vi "Do Store Reference.vi"(8 "error in (no error)":errorcluster, 10 "Store Reference Argument":T2, 11 "Data Cluster in":T1) -> (0 "error out":errorcluster, 3 "Data Cluster out":T1)   [LabVIEW 2026, in "G-AI Core.lvlib"]
uses:
  G-AI Core.lvlib
  Module Data--cluster.ctl
  Store Reference Argument--cluster.ctl
  Store Reference (Reply Payload)--cluster.ctl
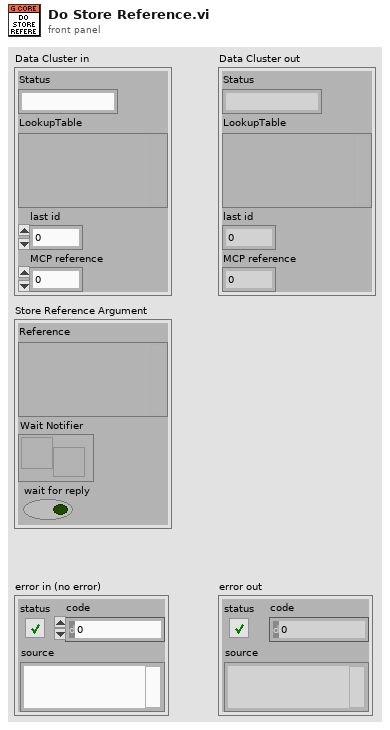
[diagram p1: front panel]
types:
  T1 = typedef "G-AI Core.lvlib/Module Data--cluster.ctl" = cluster{"Status":string, "LookupTable":variant, "last id":i32, "MCP reference":i32}
  T2 = typedef "G-AI Core.lvlib/Store Reference Argument--cluster.ctl" = cluster{"Reference":variant, "Wait Notifier":refnum<notifier>, "wait for reply":bool}
  T3 = typedef "G-AI Core.lvlib/Store Reference (Reply Payload)--cluster.ctl" = cluster{"id":string, "error":errorcluster}
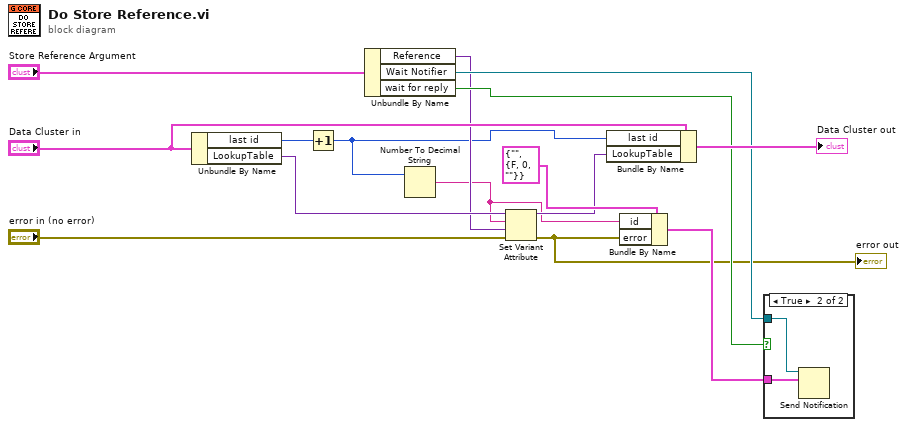
[diagram p0: block diagram]
diagram:
  n1 = Unbundle By Name("Data Cluster in") -> ("last id"=w7:i32, "LookupTable"=w6:variant)
  n2 = Increment(x=w7) -> (x+1=w3:i32)
  n3 = Unbundle By Name("Store Reference Argument") -> ("Reference"=w4:variant, "Wait Notifier"=w11:refnum<notifier>, "wait for reply"=w12:bool)
  n4 = Number To Decimal String(number=w3) -> (decimal integer string=w1:string)  [unwired: 1 in]
  n5 = Set Variant Attribute(Variant=w6, name=w1, value=w4, error in="error in (no error)") -> (Variant out=w5:variant, error out=w2:errorcluster)  [unwired: 1 out]
  "error out" <- w2
  n6 = Bundle By Name(cluster="Data Cluster in", "last id"=w3, "LookupTable"=w5) -> (→"Data Cluster out":T1)
  n7 = Bundle By Name(cluster=T3 {"id"="", "error"={"status"=FALSE, "code"=0, "source"=""}} ("Store Reference (Reply Payload)"), "id"=w1, "error"=w2) -> (w13:T3)
  n8 = case "DQMH_FIRE_NOTIFIER" shown="True" w12 {
    tunnel: w11 -> [_ w17]
    tunnel: w13 -> [_ w16]
    frame False {
    }
    frame True {
      n9 = Send Notification(notification=w16, notifier=w17) -> ()  [unwired: 1 in, 2 out]
    }
  }
